vi "SDCP BTR Encode and Decode.vi"() -> ()   [LabVIEW 2020]
uses:
  Typedefs/SDCP BTR Params.ctl
panel:
  out "BTR3 encoded":u16[](array[numeric])
  out "BTR2 encoded":u16[](array[numeric])
  out "BTR1 encoded":u16[](array[numeric])
  out "out":T1
  in  "in":T1
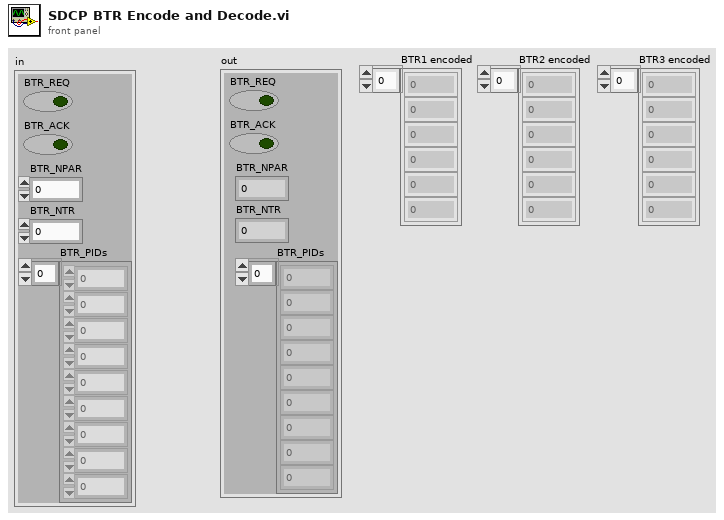
[diagram p1: front panel]
types:
  T1 = typedef "SDCP BTR Params.ctl" = cluster{"BTR_REQ":bool, "BTR_ACK":bool, "BTR_NPAR":i32, "BTR_NTR":i32, "BTR_PIDs":u8[]}
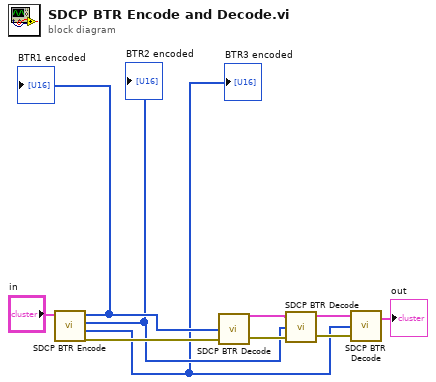
[diagram p0: block diagram]
diagram:
  n1 = call "SDCP BTR Encode.vi"("in"="in") -> ("error out"=w10:errorcluster, "BTR3 encoded"=w2:u16[], "BTR2 encoded"=w5:u16[], "BTR1 encoded"=w8:u16[])  [unwired: 3 in]
  "BTR1 encoded" <- w8
  "BTR2 encoded" <- w5
  "BTR3 encoded" <- w2
  n2 = call "SDCP BTR Decode.vi"("error in (no error)"=w10, "Frame"=w8) -> ("error out"=w7:errorcluster, "out"=w6:T1)  [unwired: 1 in]
  n3 = call "SDCP BTR Decode.vi"("error in (no error)"=w7, "Frame"=w5, "in"=w6) -> ("error out"=w4:errorcluster, "out"=w3:T1)
  n4 = call "SDCP BTR Decode.vi"("error in (no error)"=w4, "Frame"=w2, "in"=w3) -> ("out"=→"out":T1)  [unwired: 1 out]
